vi "CS_Contents_Main.vi"   [LabVIEW 2014]
doc: "This \"contents\" VI contains all components of CS, which belong to the category \"Main\". Everything in here is vital for running CS."
uses:
  CSClass/CS_Core/GUIs/GeneralObjectGUI/GeneralObjectGUI.lvlib
  CSClass/CS_Core/ObjectInspector/ObjectInspector.lvlib
  CSClass/CS_Core/CSAccessSystem/CSAccessClient/CSAccessClient.lvlib
  CSClass/CS_Core/CSAccessSystem/CSAccessViewer/CSAccessViewer.lvlib
  CSClass/CS_Core/CSSystem/CSSystemLib/CSSystemLib.lvlib
  CSClass/CS_Core/CSObj/CSObj.lvlib
  CSClass/CS_Core/BaseSM/BaseSM.lvlib
  CSClass/CS_Core/CAEObj/CAEObj.lvlib
  CSClass/CS_Core/BaseProcess/BaseProcess.lvlib
  CSClass/CS_Core/NotifierObj/NotifierObj.lvlib
  CSClass/CS_Core/SuperProc/SuperProc.lvlib
  CSClass/CS_Core/BaseGUI/BaseGUI.lvlib
  CSClass/CS_Core/GUIs/DIMGUIs/DIMHistogramGUI/DIMHistogramGUI.lvlib
  CSClass/CS_Core/GUIs/DIMGUIs/DIMTrendGUI/DIMTrendGUI.lvlib
  CSClass/CS_Core/GUIs/DIMGUIs/DIMTableView/DIMTableView.lvlib
  CSClass/CS_Core/CSTimer/CSTimer.lvlib
  CSClass/CS_Core/GUIs/CSPopUpMsgBox/CSPopUpMsgBox.lvlib
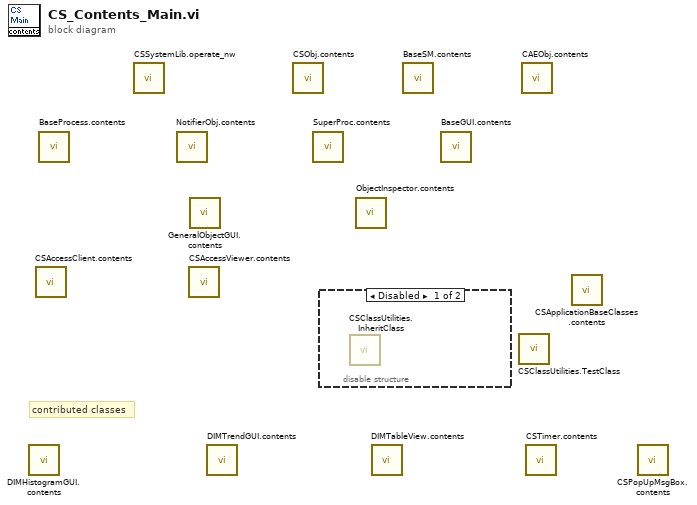
[diagram p0: block diagram]
diagram:
  # "contributed classes"
  n1 = call "DIMHistogramGUI.contents.vi"() -> ()  [unwired: 1 in]
  n2 = call "CSAccessClient.contents.vi"() -> ()  [unwired: 1 in]
  n3 = call "BaseProcess.contents.vi"() -> ()  [unwired: 1 in]
  n4 = call "CSSystemLib.operate_nw.vi"() -> ()  [unwired: 20 in]
  n5 = call "NotifierObj.contents.vi"() -> ()  [unwired: 1 in]
  n6 = call "CSAccessViewer.contents.vi"() -> ()  [unwired: 1 in]
  n7 = call "GeneralObjectGUI.contents.vi"() -> ()  [unwired: 1 in]
  n8 = call "DIMTrendGUI.contents.vi"() -> ()  [unwired: 1 in]
  n9 = call "CSObj.contents.vi"() -> ()  [unwired: 1 in]
  n10 = call "SuperProc.contents.vi"() -> ()  [unwired: 1 in]
  n11 = disable-structure shown="Disabled" {
    frame Disabled {
      n12 = call "CSClassUtilities.InheritClass.vi"() -> ()  [unwired: 1 in]
    }
    frame Enabled {
    }
  }
  n13 = call "ObjectInspector.contents.vi"() -> ()  [unwired: 1 in]
  n14 = call "DIMTableView.contents.vi"() -> ()  [unwired: 1 in]
  n15 = call "BaseSM.contents.vi"() -> ()  [unwired: 1 in]
  n16 = call "BaseGUI.contents.vi"() -> ()  [unwired: 1 in]
  n17 = call "CSClassUtilities.TestClass.vi"() -> ()  [unwired: 20 in]
  n18 = call "CAEObj.contents.vi"() -> ()  [unwired: 1 in]
  n19 = call "CSTimer.contents.vi"() -> ()  [unwired: 1 in]
  n20 = call "CSApplicationBaseClasses.contents.vi"() -> ()  [unwired: 1 in]
  n21 = call "CSPopUpMsgBox.contents.vi"() -> ()  [unwired: 1 out]
